vi "Get All Paths Helper.vi"(4 "is array element?":bool, 6 "index string":string, 8 "error in (no error)":errorcluster, 9 "parents":string[](array[string]), 10 "Variant":variant, 11 "Paths in":string[](array[string])) -> (0 "error out":errorcluster, 3 "Paths out":string[](array[string]))   [LabVIEW 2017, in "Variant Data Manipulation.lvlib"]
uses:
  Variant Data Manipulation.lvlib
  <vilib>/Utility/Data Type/NI_Data Type.lvlib
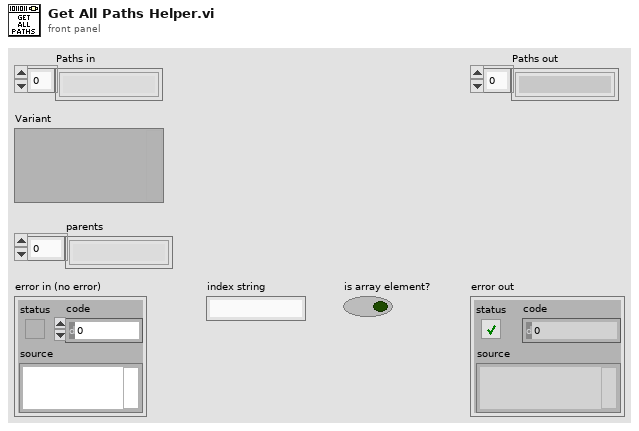
[diagram p1: front panel]
types:
  T1 = typedef "NI_Data Type.lvlib/Data Type.ctl" = enum8{"Invalid Type", "Void", "I8", "I16", "I32", "I64", "U8", "U16", "U32", "U64", "Single Float", "Double Float", "Extended Float", "Single Complex", "Double Complex", "Extended Complex", "Enum U8", "Enum U16", "Enum U32", "Enum U64", "Single Float With Unit", "Double Float With Unit", "Extended Float With Unit", "Single Complex with Unit", "Double Complex with Unit", "Extended Complex with Unit", "Boolean", "String", "Path", "Picture", "Tag", "Array", "Cluster", "Variant", "LV Variant", "Waveform", "Timestamp", "Digital Waveform", "Digital Data", "ExpressData", "Refnum", "External Data", "VI", "Poly VI", "LabVIEW Class Instance", "Fixed Point"}
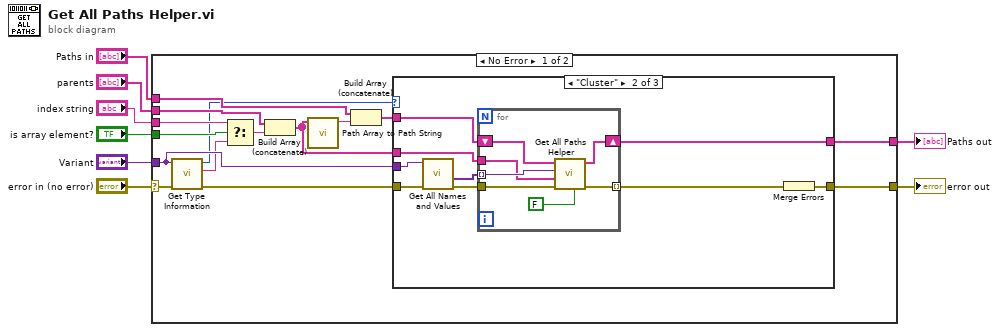
[diagram p0: block diagram]
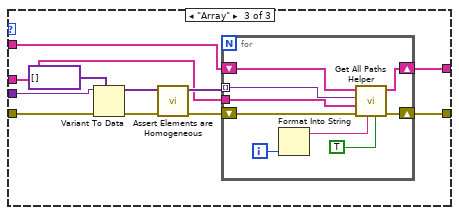
[diagram p3: hidden frame]
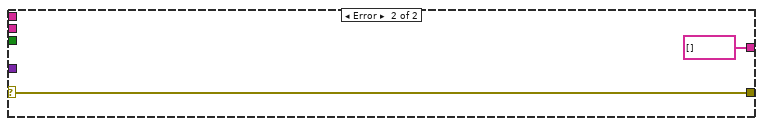
[diagram p4: hidden frame]
diagram:
  n1 = case shown="No Error" "error in (no error)" {
    selector: "error in (no error)" -> [w21 w62]
    tunnel: "Variant" -> [w22 _]
    tunnel: "is array element?" -> [w20 _]
    tunnel: "index string" -> [w19 _]
    tunnel: [w18 w62] -> w4
    tunnel: "parents" -> [w16 _]
    tunnel: "Paths in" -> [w15 _]
    tunnel: [w13 string[] []] -> w1
    frame No Error {
      n2 = call <vilib>:"Get Type Information.vi"("error in (no error)"=w21, "Variant"=w22) -> ("error out"=w23:errorcluster, "Name"=w11:string, "Type"=w12:T1)  [unwired: 5 in, 2 out]
      n3 = Select(t=w19, s=w20, f=w11) -> (s? t:f=w17:string)
      n4 = Build Array (concatenate)(w16, w17) -> (w10:string[])
      n5 = call "Path Array to Path String.vi"("path array"=w10) -> ("path"=w9:string)  [unwired: 10 in]
      n6 = Build Array (concatenate)(w15, w9) -> (w14:string[])
      n7 = case shown="\"Cluster\"" w12 {
        tunnel: w23 -> [w25 w27 w48]
        tunnel: [w25 w31 w52] -> w18
        tunnel: w22 -> [_ w34 w50]
        tunnel: w10 -> [_ w30 w44]
        tunnel: w14 -> [w24 w29 w43]
        tunnel: [w24 w28 w42] -> w13
        frame Default {
        }
        frame "Cluster" {
          n8 = call "Get All Names and Values.vi"("error in"=w27, "Cluster in"=w34) -> ("error out"=w26:errorcluster, "Values"=w33:variant[])  [unwired: 5 in, 3 out]
          n9 = for {
            tunnel: w33 -> [w41] mode=indexing
            tunnel: [w40] -> w32 mode=indexing
            shift-right: [w35] -> w28
            shift-left: w29 -> [w36]
            tunnel: w26 -> [w38]
            tunnel: w30 -> [w37]
            n10 = call "Get All Paths Helper.vi"("is array element?"=FALSE ("first call?"), "error in (no error)"=w38, "parents"=w37, "Variant"=w41, "Paths in"=w36) -> ("error out"=w40:errorcluster, "Paths out"=w35:string[])  [unwired: 5 in]
          }
          n11 = Merge Errors(w32) -> (w31:errorcluster)
        }
        frame "Array" {
          n12 = Variant To Data(error in=w48, type=variant[] [], Variant=w50) -> (data=w49:variant[], error out=w47:errorcluster)
          n13 = call "Assert Elements are Homogeneous.vi"("error in (no error)"=w47, "array in"=w49) -> ("error out"=w45:errorcluster, "array out"=w46:variant[])  [unwired: 8 in]
          n14 = for {
            tunnel: w46 -> [w58] mode=indexing
            shift-right: [w61] -> w52
            shift-left: w45 -> [w60]
            shift-right: [w54] -> w42
            shift-left: w43 -> [w53]
            tunnel: w44 -> [w55]
            i -> [w57]
            n15 = Format Into String(w57) -> (resulting string=w56:string)  [unwired: 3 in, 1 out]
            n16 = call "Get All Paths Helper.vi"("is array element?"=TRUE ("first call?"), "index string"=w56, "error in (no error)"=w60, "parents"=w55, "Variant"=w58, "Paths in"=w53) -> ("error out"=w61:errorcluster, "Paths out"=w54:string[])  [unwired: 4 in]
          }
        }
      }
    }
    frame Error {
    }
  }
  "error out" <- w4
  "Paths out" <- w1
